vi "GIF.Read.Unpack.ChangeRowLength__ogtk.vi"(9 "+1/-1 (T/F)":bool, 10 "image width":i16, 11 "Image in":u8[](array[numeric])) -> (3 "Image out":u8[](array[numeric]))   [LabVIEW 2009]
panel:
  # "GIF.Read.Unpack.ChangeRowLength.vi\n\nRe-sizes raster/rows by +/- 1 byte.\n\nPlease visit http://www.OpenG.org to learn about the\nOpen Source LabVIEW software movement.\n\nNOTICE -- YOU MUST LEAVE THIS NOTICE IN PLACE.  PER THE TERMS OF THE LICENSE BELOW, YOU MAY SUBLICENSE THIS SOFTWARE \nIN ANY WAY THAT DOES NOT CONFLICT WITH THIS LICENSE.\n\n### BSD License (http://www.opensource.org/licenses/bsd-license.php) Begin ###\n \nCopyright (c) 2007, Bill Clench <bclench@yahoo.com>\n\nAll rights reserved.\n\nRedistribution and use in source and binary forms, with or without modification, are permitted provided that the following conditions are met:\n\n    * Redistributions of source code must retain the above copyright notice, this list of conditions and the following disclaimer.\n    * Redistributions in binary form must reproduce the above copyright notice, this list of conditions and the following disclaimer in the \n       documentation and/or other materials provided with the distribution.\n    * Neither the name of SciWare, James Kring, Inc., nor the names of its contributors may be used to endorse or promote products derived \n       from this software without specific prior written permission.\n\nTHIS SOFTWARE IS PROVIDED BY THE COPYRIGHT HOLDERS AND CONTRIBUTORS \"AS IS\" AND ANY EXPRESS OR IMPLIED WARRANTIES, \nINCLUDING, BUT NOT LIMITED TO, THE IMPLIED WARRANTIES OF MERCHANTABILITY AND FITNESS FOR A PARTICULAR PURPOSE ARE \nDISCLAIMED. IN NO EVENT SHALL THE COPYRIGHT OWNER OR CONTRIBUTORS BE LIABLE FOR ANY DIRECT, INDIRECT, INCIDENTAL,\n SPECIAL, EXEMPLARY, OR CONSEQUENTIAL DAMAGES (INCLUDING, BUT NOT LIMITED TO, PROCUREMENT OF SUBSTITUTE GOODS OR \nSERVICES; LOSS OF USE, DATA, OR PROFITS; OR BUSINESS INTERRUPTION) HOWEVER CAUSED AND ON ANY THEORY OF LIABILITY, \nWHETHER IN CONTRACT, STRICT LIABILITY, OR TORT (INCLUDING NEGLIGENCE OR OTHERWISE) ARISING IN ANY WAY OUT OF THE USE \nOF THIS SOFTWARE, EVEN IF ADVISED OF THE POSSIBILITY OF SUCH DAMAGE.\n\n### BSD License End ###"
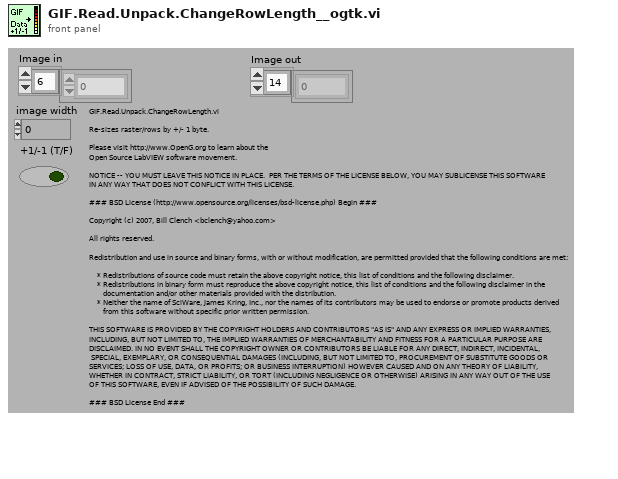
[diagram p1: front panel]
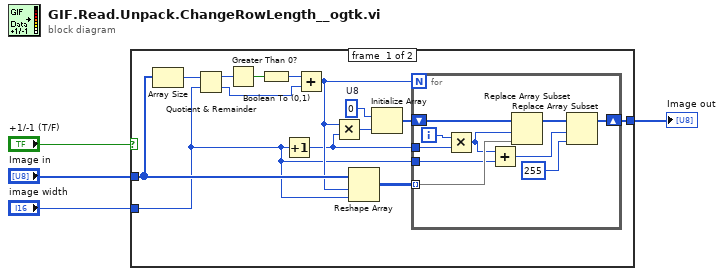
[diagram p0: block diagram]
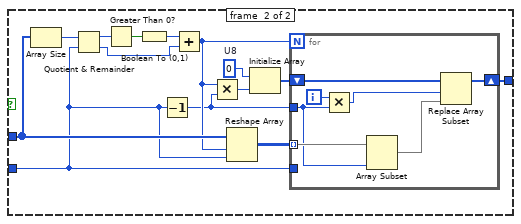
[diagram p2: hidden frame]
diagram:
  n1 = case shown="True" "+1/-1 (T/F)" {
    tunnel: "Image in" -> [w10 w34]
    tunnel: "image width" -> [w5 w29]
    tunnel: [w6 w30] -> w2
    frame #0 {
      w11 = u8 0  # U8
      n2 = Array Size(array=w10) -> (size(s)=w13:i32)
      n3 = Quotient & Remainder(x=w13, y=w5) -> (x-y*floor(x/y)=w17:i32, floor(x/y)=w14:i32)
      n4 = Greater Than 0?(x=w17) -> (x > 0?=w16:bool)
      n5 = Boolean To (0,1)(Boolean=w16) -> (0, 1=w15:i16)
      n6 = Increment(x=w5) -> (x+1=w7:i16)
      n7 = Add(x=w15, y=w14) -> (x+y=w9:i32)
      n8 = Multiply(x=w9, y=w7) -> (x*y=w12:i32)
      n9 = Reshape Array(w10, w9, w5) -> (w8:u8[][])
      n10 = Initialize Array(w11, w12) -> (w18:u8[])
      n11 = for {
        N: w9 -> [_]
        shift-right: [w24] -> w6
        shift-left: w18 -> [w28]
        tunnel: w7 -> [w27]
        tunnel: w8 -> [w23] mode=indexing
        tunnel: w5 -> [w19]
        i -> [w26]
        n12 = Multiply(x=w26, y=w27) -> (x*y=w21:i32)
        n13 = Add(x=w21, y=w19) -> (x+y=w20:i32)
        n14 = Replace Array Subset(array=w28, new element=w23, index=w21) -> (w25:u8[])
        n15 = Replace Array Subset(array=w25, new element=u8 255 ("new element/subarray"), index=w20) -> (w24:u8[])
      }
    }
    frame #1 {
      w35 = u8 0  # U8
      n16 = Array Size(array=w34) -> (size(s)=w37:i32)
      n17 = Quotient & Remainder(x=w37, y=w29) -> (x-y*floor(x/y)=w41:i32, floor(x/y)=w38:i32)
      n18 = Greater Than 0?(x=w41) -> (x > 0?=w40:bool)
      n19 = Boolean To (0,1)(Boolean=w40) -> (0, 1=w39:i16)
      n20 = Decrement(x=w29) -> (x-1=w31:i16)
      n21 = Add(x=w39, y=w38) -> (x+y=w33:i32)
      n22 = Multiply(x=w33, y=w31) -> (x*y=w36:i32)
      n23 = Reshape Array(w34, w33, w29) -> (w32:u8[][])
      n24 = Initialize Array(w35, w36) -> (w42:u8[])
      n25 = for {
        N: w33 -> [_]
        shift-right: [w46] -> w30
        shift-left: w42 -> [w49]
        tunnel: w31 -> [w44]
        tunnel: w32 -> [w45] mode=indexing
        tunnel: w29 -> [_]
        i -> [w48]
        n26 = Multiply(x=w48, y=w44) -> (x*y=w47:i32)
        n27 = Array Subset(array=w45, length=w44) -> (w43:u8[])  [unwired: 1 in]
        n28 = Replace Array Subset(array=w49, new element=w43, index=w47) -> (w46:u8[])
      }
    }
  }
  "Image out" <- w2
